vi "prima_apl_v2.vi"() -> ()   [LabVIEW 2009]
panel:
  out "Terminal de tip Numeric":i16
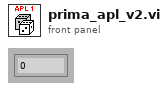
[diagram p1: front panel]
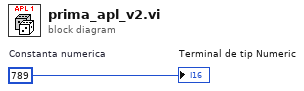
[diagram p0: block diagram]
diagram:
  w1 = 789  # Constanta numerica
  "Terminal de tip Numeric" <- w1
